vi "SWERV_ODOM_ABS_ACQUIRE.vi"(9 "in Swerve Module Positions":T6[](array[typedef]) {"Angle"."SIN" format="%13.4f"; "Angle"."COS" format="%13.4f"; "Angle"."VALUE" format="%13.4f"}, 10 "Gyro_Heading_Rad":dbl, 11 "in SWERVE_DRIVE_KINEMATICS":T1 {"SavedModuleStates"."Angle"."SIN" format="%13.4f"; "SavedModuleStates"."Angle"."COS" format="%13.4f"; "SavedModuleStates"."Angle"."VALUE" format="%13.4f"; "PrevCoR"."Y" format="%14.3f"; "PrevCoR"."X" format="%14.3f"; "Modules"."Y" format="%14.3f"; "Modules"."X" format="%14.3f"}) -> ()   [LabVIEW 2019]
uses:
  <vilib>/Rock Robotics/WPI/ThirdParty/JAS_Junk/TrajLib/TypeDef/SWERVE_DRIVE_MODULE_POSITION.ctl
  <vilib>/Rock Robotics/WPI/ThirdParty/JAS_Junk/TrajLib/TypeDef/ROTATION2D.ctl
  <vilib>/Rock Robotics/WPI/ThirdParty/JAS_Junk/TrajLib/TypeDef/SWERVE_DRIVE_KINEMATICS.ctl
  <vilib>/Analysis/Matrix/Datatypes/RealMatrix.ctl
  <vilib>/Rock Robotics/WPI/ThirdParty/JAS_Junk/TrajLib/TypeDef/TRANSLATION2D.ctl
  <vilib>/Rock Robotics/WPI/ThirdParty/JAS_Junk/TrajLib/TypeDef/SWERVE_DRIVE_MODULE_STATE.ctl
  <vilib>/Rock Robotics/WPI/ThirdParty/JAS_Junk/TrajLib/Trajectory_Library.lvlib
  <vilib>/Analysis/Matrix/NI_Matrix.lvlib
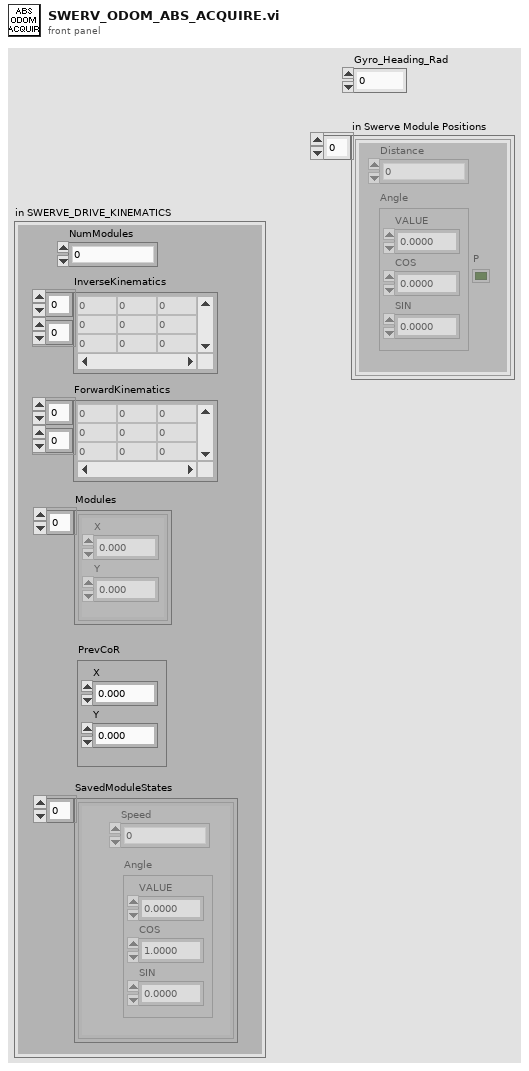
[diagram p1: front panel]
types:
  T1 = typedef "Trajectory_Library.lvlib/SWERVE_DRIVE_KINEMATICS.ctl" = cluster{"NumModules":i32, "InverseKinematics":T2, "ForwardKinematics":T2, "Modules":T3[], "PrevCoR":T3, "SavedModuleStates":T4[]}
  T2 = typedef "NI_Matrix.lvlib/RealMatrix.ctl" = dbl[][]
  T3 = typedef "Trajectory_Library.lvlib/TRANSLATION2D.ctl" = cluster{"X":dbl, "Y":dbl}
  T4 = typedef "Trajectory_Library.lvlib/SWERVE_DRIVE_MODULE_STATE.ctl" = cluster{"Speed":dbl, "Angle":T5}
  T5 = typedef "Trajectory_Library.lvlib/ROTATION2D.ctl" = cluster{"VALUE":dbl, "COS":dbl, "SIN":dbl}
  T6 = typedef "Trajectory_Library.lvlib/SWERVE_DRIVE_MODULE_POSITION.ctl" = cluster{"Distance":dbl, "Angle":T5, "P":bool}
  T7 = typedef "Trajectory_Library.lvlib/SWERVE_DRIVE_ODOMETRY.ctl" = cluster{"POSE":T8, "GyroOffset":T5, "PreviousAngle":T5, "PrevModulePositions":T6[], "NumModules":i32}
  T8 = typedef "Trajectory_Library.lvlib/POSE2D.ctl" = cluster{"TRANSLATION":T3, "ROTATION":T5}
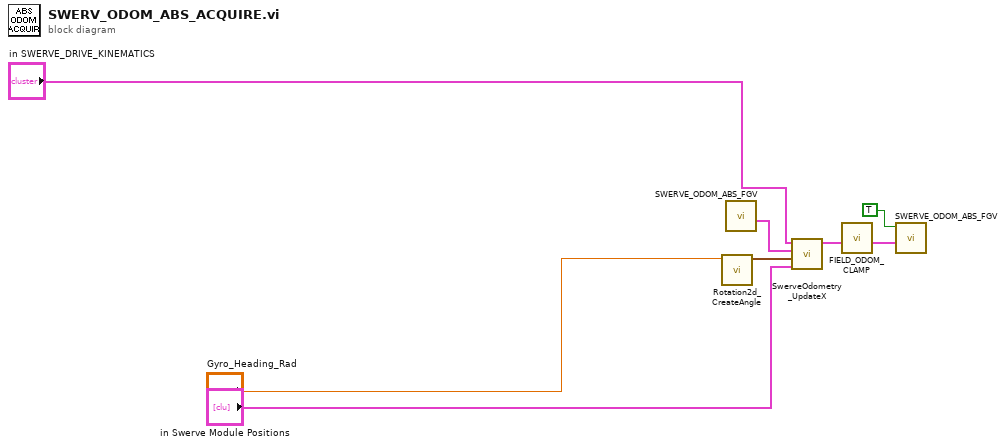
[diagram p0: block diagram]
diagram:
  n1 = call <vilib>:"Rotation2d_CreateAngle.vi"("Angle"="Gyro_Heading_Rad") -> ("ROTATION"=w6:T5)  [unwired: 10 in]
  n2 = call "SWERVE_ODOM_ABS_FGV.vi"() -> ("out SWERVE_DRIVE_ODOMETRY"=w5:T7)  [unwired: 11 in]
  n3 = call <vilib>:"SwerveOdometry_UpdateX.vi"("module Positions"="in Swerve Module Positions", "gyroAngle"=w6, "in SWERVE_DRIVE_ODOMETRY"=w5, "SWERVE_DRIVE_KINEMATICS"="in SWERVE_DRIVE_KINEMATICS") -> ("out SWERVE_DRIVE_ODOMETRY"=w2:T7)  [unwired: 5 in, 2 out]
  n4 = call "FIELD_ODOM_CLAMP.vi"("in SWERVE_DRIVE_ODOMETRY"=w2) -> ("out SWERVE_DRIVE_ODOMETRY"=w3:T7)  [unwired: 10 in]
  n5 = call "SWERVE_ODOM_ABS_FGV.vi"("in SWERVE_DRIVE_ODOMETRY"=w3, "WRITE"=TRUE) -> ()  [unwired: 9 in, 1 out]
